vi "NumericLimitTest.vi"(11 "Numeric":dbl) -> (0 "error out":errorcluster, 2 "Report Text":string, 3 "Numeric Measurement":dbl)   [LabVIEW 2020]
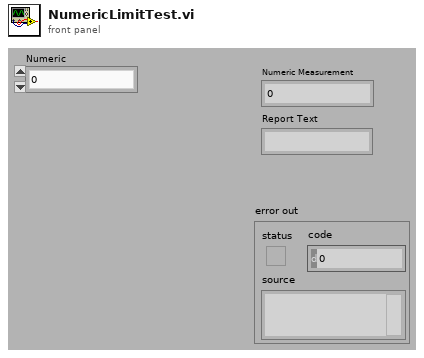
[diagram p1: front panel]
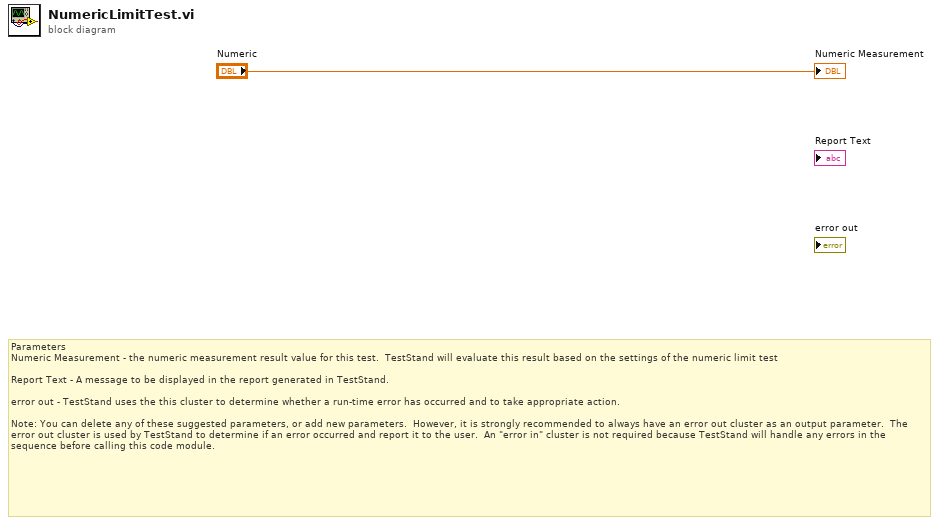
[diagram p0: block diagram]
diagram:
  # "Parameters\nNumeric Measurement - the numeric measurement result value for this test.  TestStand will evaluate this result based on the settings of the numeric limit test\n\nReport Text - A message to be displayed in the report generated in TestStand. \n\nerror out - TestStand uses the this cluster to determine whether a run-time error has occurred and to take appropriate action.  \n\nNote: You can delete any of these suggested parameters, or add new parameters.  However, it is strongly recommended to always have an error out cluster as an output parameter.  The error out cluster is used by TestStand to determine if an error occurred and report it to the user.  An \"error in\" cluster is not required because TestStand will handle any errors in the sequence before calling this code module."
  "Numeric Measurement" <- "Numeric"
